vi "oa_Get DSA 447x Oversample Rate and Filter Delay.vi"(9 "EAR enabled? (F)":bool, 11 "vibration signal sample rate":dbl) -> (1 "start":dbl, 3 "oversample rate":dbl format="%#_6f")   [LabVIEW 2017, in "SoundVib_TachProcess.lvlib"]
uses:
  <vilib>/addons/Sound and Vibration/Order Analysis/Tach Process/SoundVib_TachProcess.lvlib
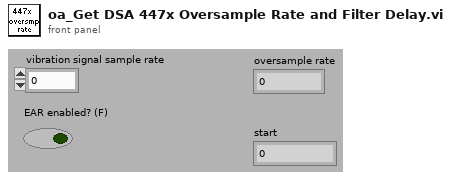
[diagram p1: front panel]
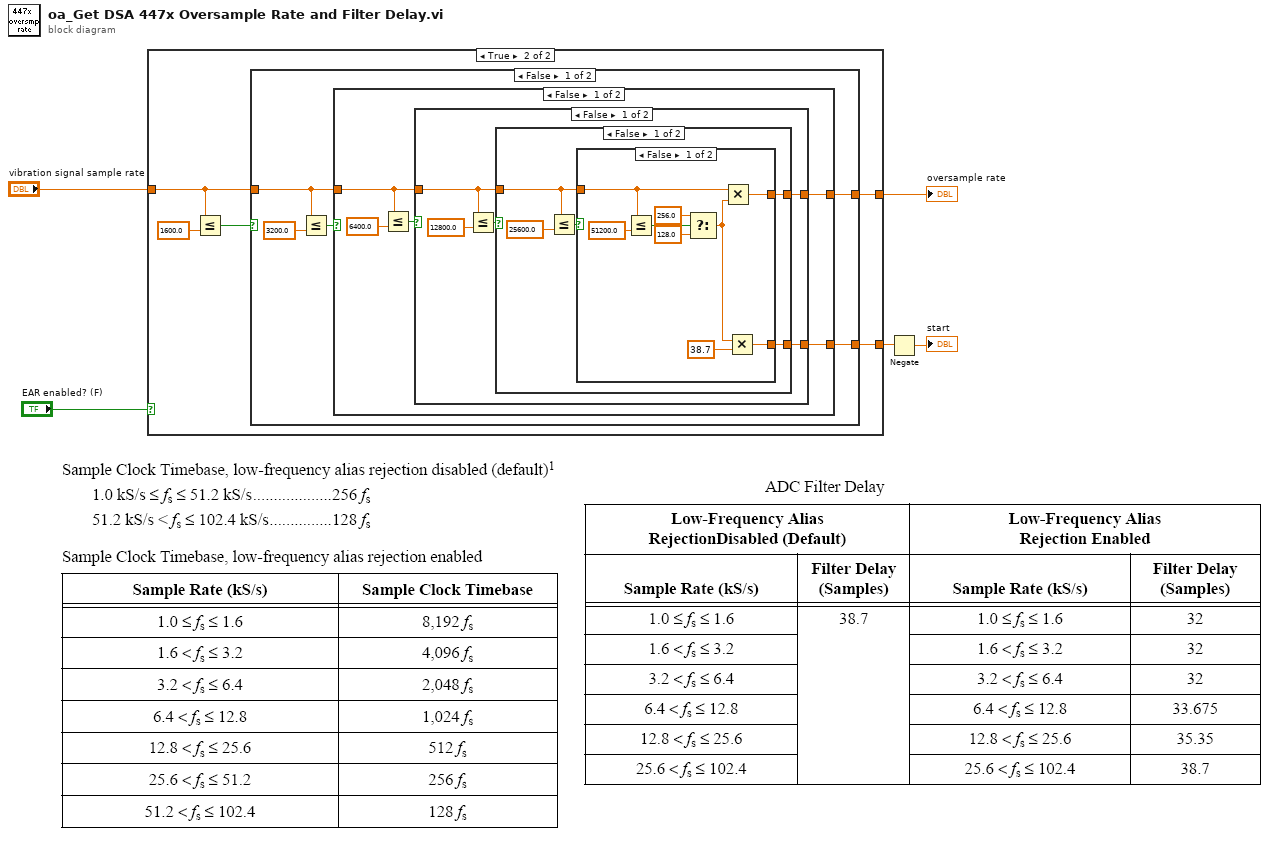
[diagram p0: block diagram]
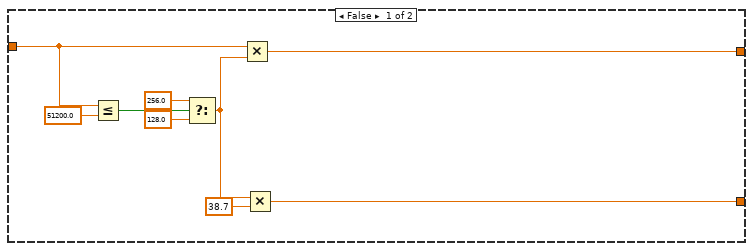
[diagram p2: hidden frame]
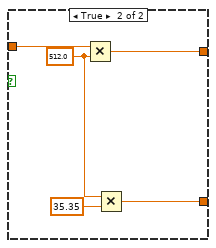
[diagram p3: hidden frame]
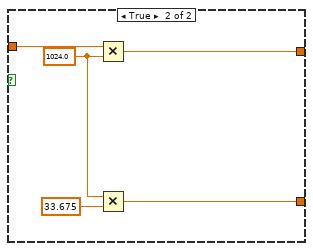
[diagram p4: hidden frame]
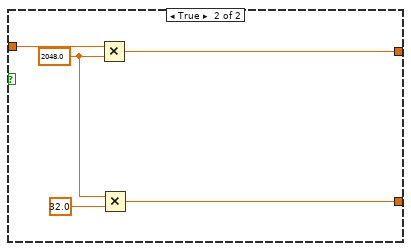
[diagram p5: hidden frame]
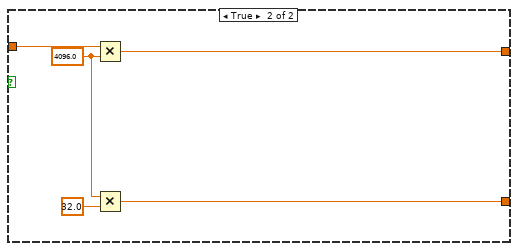
[diagram p6: hidden frame]
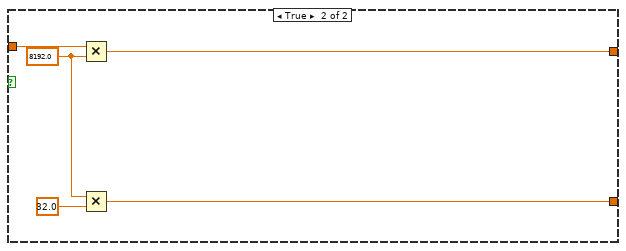
[diagram p7: hidden frame]
diagram:
  n1 = case shown="True" "EAR enabled? (F)" {
    tunnel: "vibration signal sample rate" -> [w8 w17]
    tunnel: [w9 w15] -> w2
    tunnel: [w6 w16] -> w3
    frame False {
      n2 = Less Or Equal?(x=w8, y=51200.0) -> (x <= y?=w13:bool)
      n3 = Select(t=256.0, s=w13, f=128.0) -> (s? t:f=w7:dbl)
      n4 = Multiply(x=w8, y=w7) -> (x*y=w6:dbl)
      n5 = Multiply(x=w7, y=38.7) -> (x*y=w9:dbl)
    }
    frame True {
      n6 = Less Or Equal?(x=w17, y=1600.0) -> (x <= y?=w18:bool)
      n7 = case shown="False" w18 {
        tunnel: w17 -> [w22 w73]
        tunnel: [w21 w72] -> w16
        tunnel: [w20 w69] -> w15
        frame False {
          n8 = Less Or Equal?(x=w22, y=3200.0) -> (x <= y?=w23:bool)
          n9 = case shown="False" w23 {
            tunnel: w22 -> [w27 w68]
            tunnel: [w26 w67] -> w21
            tunnel: [w25 w64] -> w20
            frame False {
              n10 = Less Or Equal?(x=w27, y=6400.0) -> (x <= y?=w28:bool)
              n11 = case shown="False" w28 {
                tunnel: w27 -> [w32 w63]
                tunnel: [w31 w61] -> w26
                tunnel: [w30 w59] -> w25
                frame False {
                  n12 = Less Or Equal?(x=w32, y=12800.0) -> (x <= y?=w33:bool)
                  n13 = case shown="False" w33 {
                    tunnel: w32 -> [w37 w58]
                    tunnel: [w36 w57] -> w31
                    tunnel: [w35 w54] -> w30
                    frame False {
                      n14 = Less Or Equal?(x=w37, y=25600.0) -> (x <= y?=w38:bool)
                      n15 = case shown="False" w38 {
                        tunnel: w37 -> [w43 w53]
                        tunnel: [w44 w52] -> w36
                        tunnel: [w41 w49] -> w35
                        frame False {
                          n16 = Less Or Equal?(x=w43, y=51200.0) -> (x <= y?=w47:bool)
                          n17 = Select(t=256.0, s=w47, f=128.0) -> (s? t:f=w42:dbl)
                          n18 = Multiply(x=w43, y=w42) -> (x*y=w44:dbl)
                          n19 = Multiply(x=w42, y=38.7) -> (x*y=w41:dbl)
                        }
                        frame True {
                          w51 = 512.0 ("y")
                          n20 = Multiply(x=w53, y=w51) -> (x*y=w52:dbl)
                          n21 = Multiply(x=w51, y=35.35) -> (x*y=w49:dbl)
                        }
                      }
                    }
                    frame True {
                      w56 = 1024.0 ("y")
                      n22 = Multiply(x=w58, y=w56) -> (x*y=w57:dbl)
                      n23 = Multiply(x=w56, y=33.675) -> (x*y=w54:dbl)
                    }
                  }
                }
                frame True {
                  w60 = 2048.0 ("y")
                  n24 = Multiply(x=w63, y=w60) -> (x*y=w61:dbl)
                  n25 = Multiply(x=w60, y=32.0) -> (x*y=w59:dbl)
                }
              }
            }
            frame True {
              w66 = 4096.0 ("y")
              n26 = Multiply(x=w68, y=w66) -> (x*y=w67:dbl)
              n27 = Multiply(x=w66, y=32.0) -> (x*y=w64:dbl)
            }
          }
        }
        frame True {
          w71 = 8192.0 ("y")
          n28 = Multiply(x=w73, y=w71) -> (x*y=w72:dbl)
          n29 = Multiply(x=w71, y=32.0) -> (x*y=w69:dbl)
        }
      }
    }
  }
  "oversample rate" <- w3
  n30 = Negate(x=w2) -> (-x=→"start":dbl)
